vi "Git sandbox.vi"() -> ()   [LabVIEW 2019, in "Git.lvclass"]
uses:
  Git.lvclass
  Git.lvclass/Git.ctl
panel:
  in  "Option":string(combo)="start"
  in  "Command":string(combo)="config"
  out "return code":i32
  out "standard error":string
  out "standard output":string="git flow init -d"
  in  "Repository Path":path=path "C:/Users/patrick/Documents/GitHub/Oxford-1820"
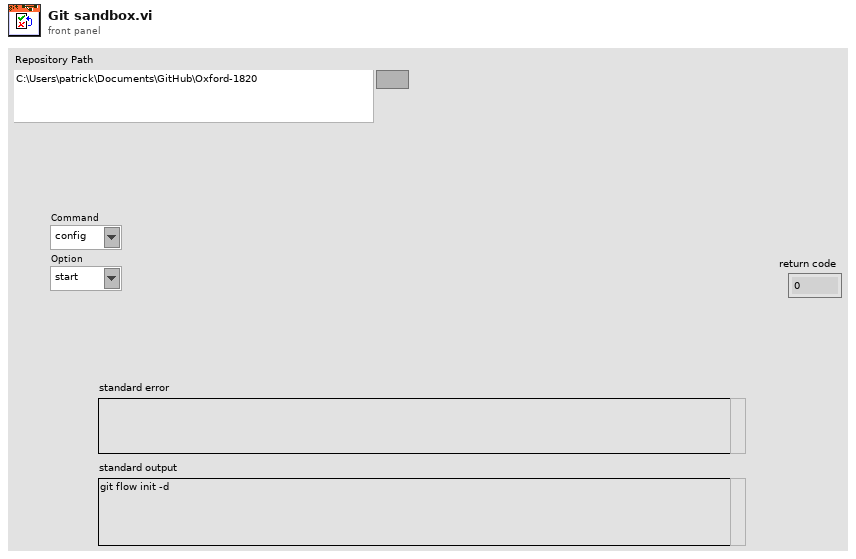
[diagram p1: front panel]
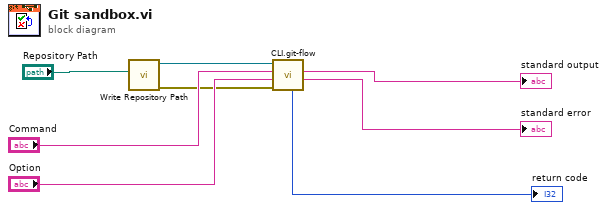
[diagram p0: block diagram]
diagram:
  n1 = call "Write Repository Path.vi"("Repository Path"="Repository Path") -> ("error out"=w4:errorcluster, "Git out"=w5:refnum<class "Git.lvclass">)  [unwired: 9 in]
  n2 = call "CLI.git-flow.vi"("error in (no error)"=w4, "Branch"="Option", "Command"="Command", "Git in"=w5) -> ("standard error"=→"standard error":string, "standard output"=→"standard output":string, "return code"=→"return code":i32)  [unwired: 3 in, 2 out]
